vi "Launcher.vi"() -> ()   [LabVIEW 2021]
uses:
  Controls/Mainctrl.ctl
panel:
  in  "Cancel Button":bool
  in  "Agua Cl":bool
  in  "Calorimetria":bool
  in  "Entalpia Reacción":bool
  in  "Calentador Tf":bool
  in  "Calentador Q":bool
  in  "Vaporizador":bool
  # "INSTITUCIÓN UNIVERSITARIA POLITÉCNICO GRANCOLOMBIANO\nTHERMO BASICS"
  # "Seleccione la práctica a realizar:"
  # "Desarrollado por:\n     Semillero Electroquimica e Innovación Ambiental - SEIA"
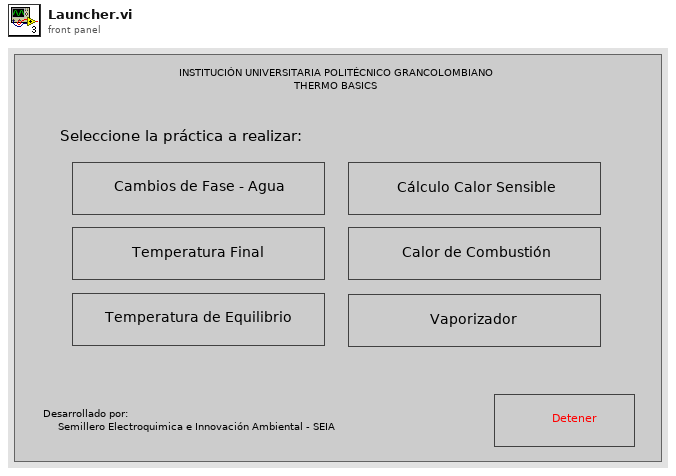
[diagram p1: front panel]
types:
  T1 = typedef "Mainctrl.ctl" = enum16{"Now?", "Vaporizador", "Agua_CL", "Sensible Q", "Sensible Tf", "Equilibrio", "Reacción", "Stop"}
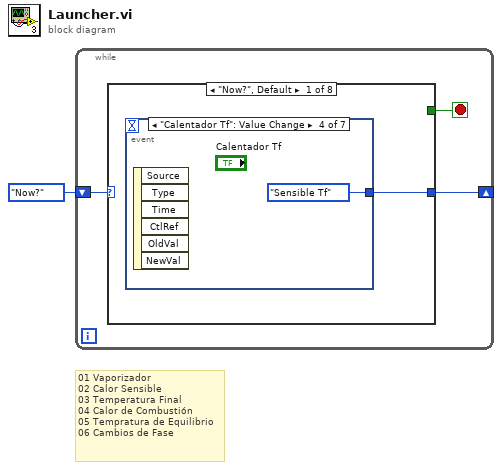
[diagram p0: block diagram]
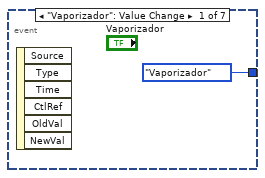
[diagram p2: hidden frame]
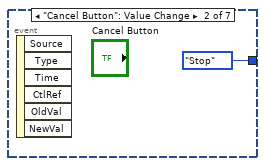
[diagram p3: hidden frame]
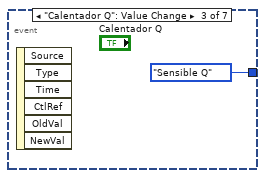
[diagram p4: hidden frame]
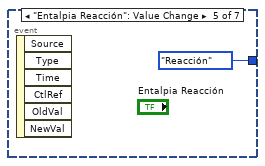
[diagram p5: hidden frame]
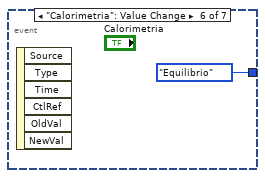
[diagram p6: hidden frame]
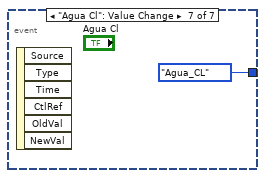
[diagram p7: hidden frame]
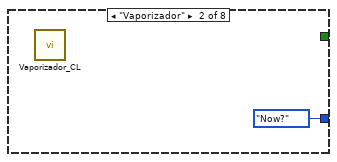
[diagram p8: hidden frame]
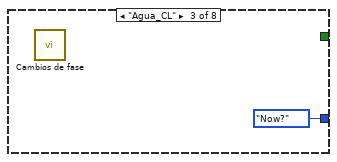
[diagram p9: hidden frame]
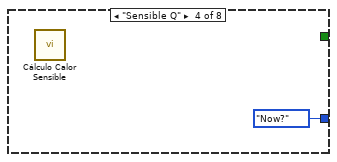
[diagram p10: hidden frame]
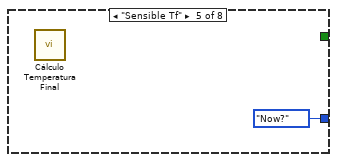
[diagram p11: hidden frame]
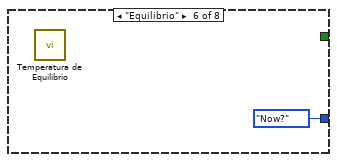
[diagram p12: hidden frame]
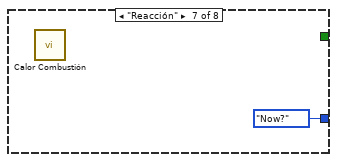
[diagram p13: hidden frame]
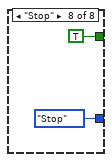
[diagram p14: hidden frame]
diagram:
  # "01 Vaporizador\n02 Calor Sensible\n03 Temperatura Final\n04 Calor de Combustión\n05 Tempratura de Equilibrio\n06 Cambios de Fase"
  n1 = while {
    shift-right: [w3] -> _
    shift-left: Mainctrl."Now?" -> [w4]
    stop <- w2 stop-if-true
    n2 = case shown="\"Now?\", Default" w4 {
      tunnel: [w5 Mainctrl."Now?" Mainctrl."Now?" Mainctrl."Now?" Mainctrl."Now?" Mainctrl."Now?" Mainctrl."Now?" Mainctrl."Stop"] -> w3
      tunnel: [_ _ _ _ _ _ _ TRUE] -> w2
      frame "Now?", Default {
        n3 = event shown="[3] \"Calentador Tf\": Value Change" {
          selector: _ -> [_ _ _ _ _ _ _]
          dyn-events: _ -> [_ _ _ _ _ _ _]
          timeout: _ -> [_ _ _ _ _ _ _]
          tunnel: [Mainctrl."Vaporizador" Mainctrl."Stop" Mainctrl."Sensible Q" Mainctrl."Sensible Tf" Mainctrl."Reacción" Mainctrl."Equilibrio" Mainctrl."Agua_CL"] -> w5
          event "Vaporizador": Value Change {
            n4 = event-data() -> ()  [unwired: 1 in, 6 out]
          }
          event "Cancel Button": Value Change {
            n5 = event-data() -> ()  [unwired: 1 in, 6 out]
          }
          event "Calentador Q": Value Change {
            n6 = event-data() -> ()  [unwired: 1 in, 6 out]
          }
          event "Calentador Tf": Value Change {
            n7 = event-data() -> ()  [unwired: 1 in, 6 out]
          }
          event "Entalpia Reacción": Value Change {
            n8 = event-data() -> ()  [unwired: 1 in, 6 out]
          }
          event "Calorimetria": Value Change {
            n9 = event-data() -> ()  [unwired: 1 in, 6 out]
          }
          event "Agua Cl": Value Change {
            n10 = event-data() -> ()  [unwired: 1 in, 6 out]
          }
        }
      }
      frame "Vaporizador" {
        n11 = call "Vaporizador_CL.vi"() -> ()  [unwired: 12 in]
      }
      frame "Agua_CL" {
        n12 = call "Cambios de fase.vi"() -> ()  [unwired: 12 in]
      }
      frame "Sensible Q" {
        n13 = call "Cálculo Calor Sensible.vi"() -> ()  [unwired: 12 in]
      }
      frame "Sensible Tf" {
        n14 = call "Cálculo Temperatura Final.vi"() -> ()  [unwired: 12 in]
      }
      frame "Equilibrio" {
        n15 = call "Temperatura de Equilibrio.vi"() -> ()  [unwired: 12 in]
      }
      frame "Reacción" {
        n16 = call "Calor Combustión.vi"() -> ()  [unwired: 12 in]
      }
      frame "Stop" {
      }
    }
  }
